vi "LV_n_UDP_clients.vi"() -> ()   [LabVIEW 2020]
panel:
  in  "Open Multi Ports":bool
  in  "Send Test Image":bool
  in  "h":i32=10 min=1 max=5000 step=1
  in  "w":i32=1 min=1 max=5000 step=1
  out "Elaps ms":u32
  in  "Send Image":bool
  out "Path to Python script":path
  in  "Stop":bool
  out "Answer":string
  in  "Ping":bool
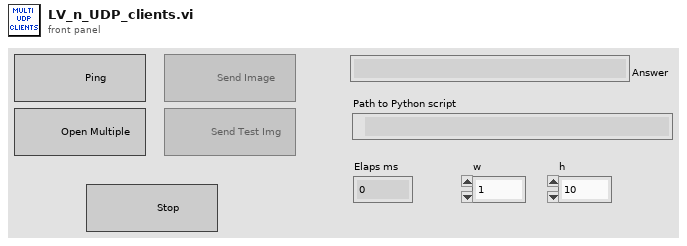
[diagram p1: front panel]
types:
  T1 = enum8{"Enabled", "Disabled", "Disabled and Grayed Out"}
  T2 = typedef "Image Type" = u32
  T3 = typedef "IMAQ Image.ctl" = refnum<image>
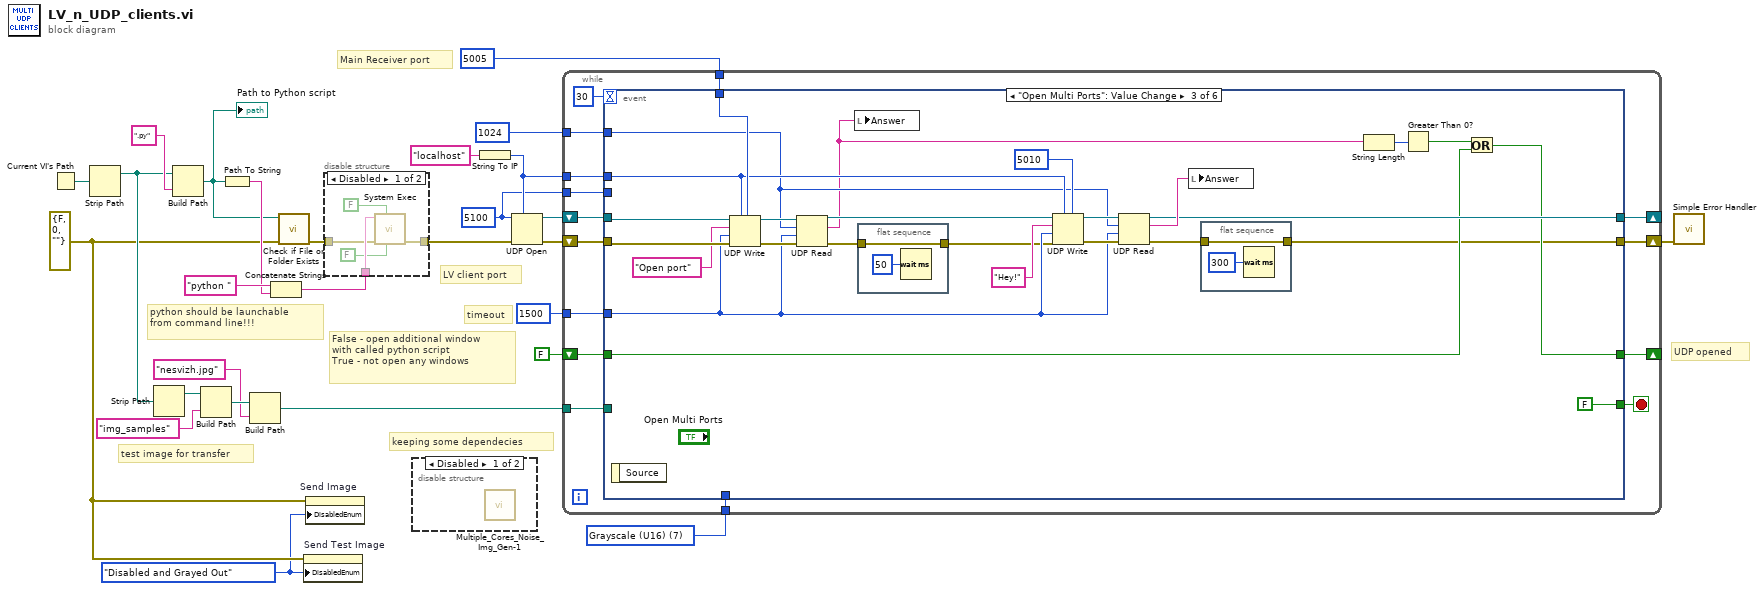
[diagram p0: block diagram]
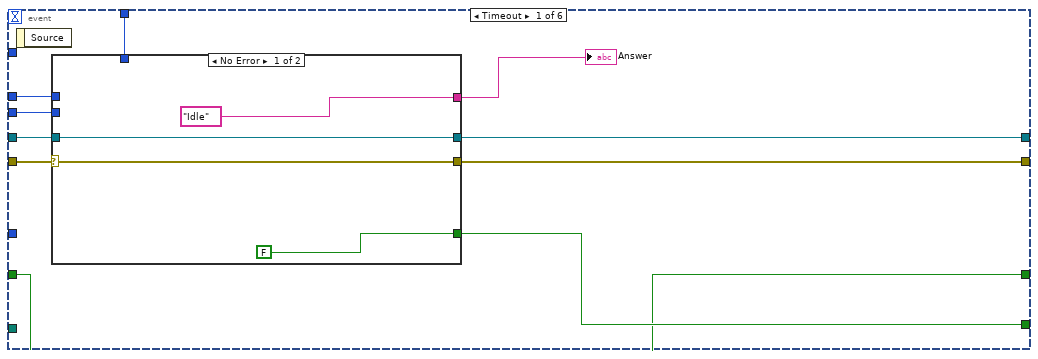
[diagram p4: hidden frame]
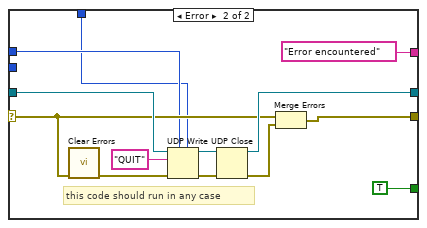
[diagram p5: hidden frame]
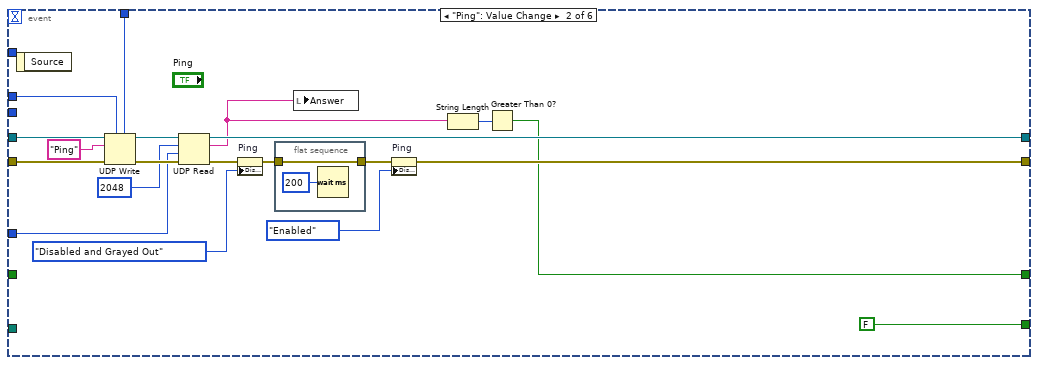
[diagram p6: hidden frame]
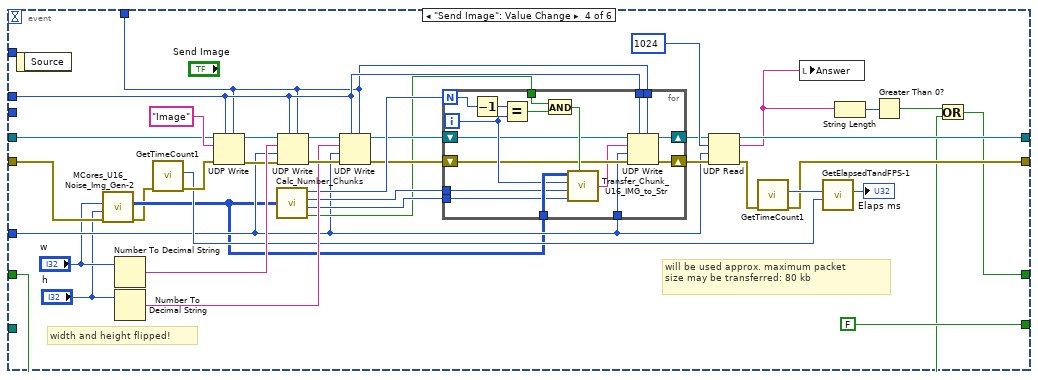
[diagram p7: hidden frame]
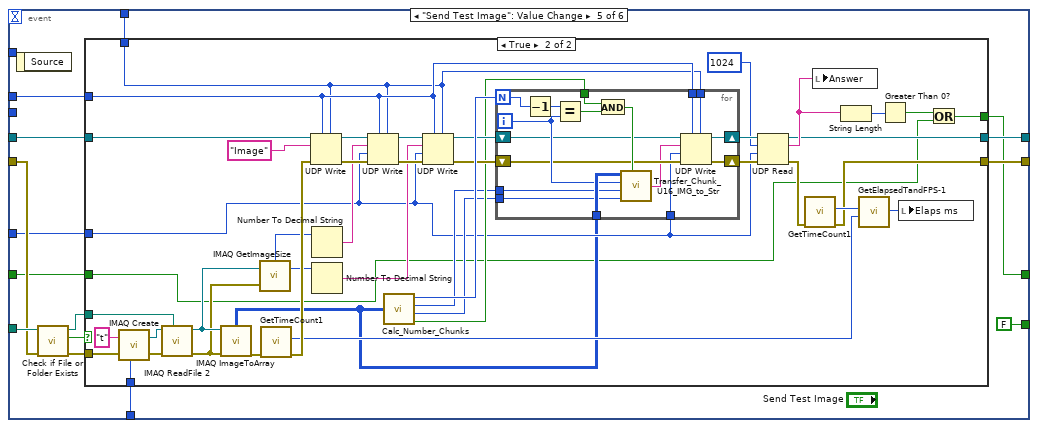
[diagram p8: hidden frame]
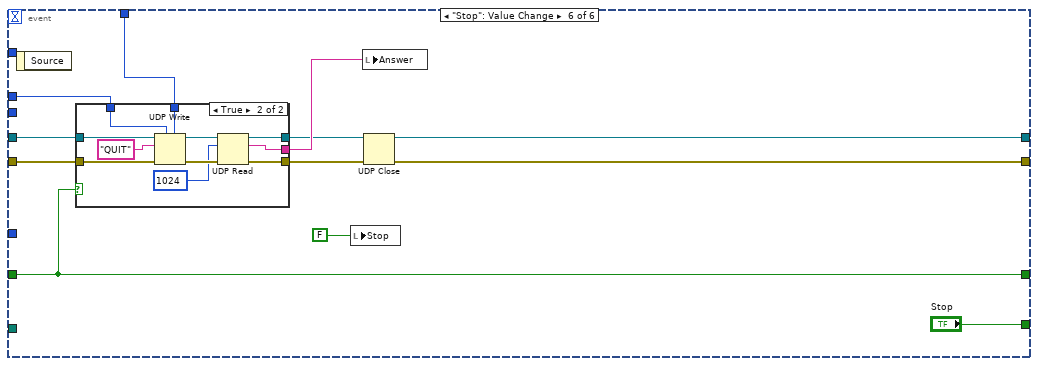
[diagram p10: hidden frame]
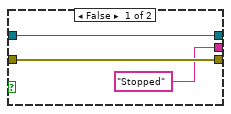
[diagram p11: hidden frame]
diagram:
  w3 = T1."Disabled and Grayed Out" ("Disabled")
  w5 = T2 7 items=["Grayscale (U8)", "Grayscale (I16)", "Grayscale (SGL)", "Complex (CSG)", "RGB (U32)", "HSL (U32)", "RGB (U64)", "Grayscale (U16)"] ("Image Type")
  w14 = u16 5100 ("remote port or service name")
  w4 = errorcluster {"status"=FALSE, "code"=0, "source"=""} ("error in (no error)")
  # "UDP opened"
  # "test image for transfer"
  # "keeping some dependecies"
  # "timeout"
  # "Main Receiver port"
  # "LV client port"
  # "False - open additional window\nwith called python script\nTrue - not open any windows"
  # "python should be launchable \nfrom command line!!!"
  n1 = Current VI's Path() -> (path=w26:path)
  n2 = Strip Path(path=w26) -> (stripped path=w11:path)  [unwired: 1 out]
  n3 = Strip Path(path=w11) -> (stripped path=w10:path)  [unwired: 1 out]
  n4 = Build Path(base path=w11, name or relative path=".py" ("string")) -> (appended path=w21:path)
  "Path to Python script" <- w21
  n5 = Build Path(base path=w10, name or relative path="img_samples" ("string")) -> (appended path=w8:path)
  n6 = Path To String(path=w21) -> (string=w22:string)
  n7 = Build Path(base path=w8, name or relative path="nesvizh.jpg" ("string")) -> (appended path=w6:path)
  n8 = Concatenate Strings("python " ("command line"), w22) -> (w24:string)
  n9 = call <vilib>:"Check if File or Folder Exists.vi"("error in (no error)"=w4, "path"=w21) -> ("error out"=w20:errorcluster)  [unwired: 7 in, 2 out]
  n10 = property on="Send Test Image" class="Bool"(error in=w4, "DisabledEnum"=w3) -> ()  [unwired: 1 in, 2 out]
  n11 = property on="Send Image" class="Bool"(error in=w4, "DisabledEnum"=w3) -> ()  [unwired: 1 in, 2 out]
  n12 = disable-structure shown="Disabled" {
    disable-tunnel: w24 -> [w32 _]
    disable-tunnel: [w31 w33] -> w19
    disable-tunnel: w20 -> [w29 w33]
    frame Disabled {
      n13 = call <vilib>:"System Exec.vi"("run minimized? (F)"=FALSE, "wait until completion? (T)"=FALSE, "error in (no error)"=w29, "command line"=w32) -> ("error out"=w31:errorcluster)  [unwired: 4 in, 3 out]
    }
    frame Enabled {
    }
  }
  n14 = disable-structure shown="Disabled" {
    frame Disabled {
      n15 = call "Multiple_Cores_Noise_Img_Gen-1.vi"() -> ()  [unwired: 10 in, 2 out]
    }
    frame Enabled {
    }
  }
  n16 = String To IP(1:"localhost" ("address")) -> (0:w15:u32)
  n17 = UDP Open(7:w15, 8:w19, 11:w14) -> (port=w17:refnum<k16>, 0:w18:errorcluster)  [unwired: 2 in, 1 out]
  n18 = while {
    shift-right: [w45] -> _
    shift-left: w17 -> [w46]
    shift-right: [w43] -> w27
    shift-left: w18 -> [w47]
    tunnel: w15 -> [w41]
    tunnel: w14 -> [w42]
    tunnel: u16 5005 ("remote port or service name") -> [w40]
    tunnel: 1500 -> [w39]
    tunnel: w6 -> [w38]
    tunnel: w5 -> [w37]
    shift-right: [w35] -> _
    shift-left: FALSE -> [w36]
    tunnel: 1024 -> [w34]
    stop <- w44 stop-if-true
    n19 = event shown="[2] \"Open Multi Ports\": Value Change" {
      selector: _ -> [_ _ _ _ _ _]
      dyn-events: _ -> [_ _ _ _ _ _]
      timeout: 30 -> [_ _ _ _ _ _]
      tunnel: [w54 FALSE ("Stop") FALSE ("Stop") FALSE ("Stop") FALSE ("Stop") "Stop"] -> w44
      tunnel: w47 -> [w58 w89 w123 w137 w195 w268]
      tunnel: w46 -> [w57 w88 w122 w164 w190 w269]
      tunnel: [w56 w84 w108 w158 w185 w270] -> w45
      tunnel: [w55 w91 w100 w150 w186 w271] -> w43
      tunnel: w42 -> [w52 _ _ _ _ _]
      tunnel: w41 -> [w51 w81 w116 w139 w189 w264]
      tunnel: w40 -> [w50 w80 w120 w138 w188 w263]
      tunnel: w39 -> [_ w79 w111 w140 w187 _]
      tunnel: w38 -> [_ _ _ _ w196 _]
      tunnel: w37 -> [_ _ _ _ w191 _]
      tunnel: w36 -> [w49 _ w105 w129 w183 w262]
      tunnel: [w49 w76 w103 w128 w184 w262] -> w35
      tunnel: w34 -> [_ _ w110 _ _ _]
      event Timeout {
        n20 = event-data() -> ()  [unwired: 1 in, 1 out]
        n21 = case shown="No Error" w58 {
          selector: w58 -> [w61 w70]
          tunnel: [w62 w73] -> w56
          tunnel: w57 -> [w62 w72]
          tunnel: [w61 w71] -> w55
          tunnel: [FALSE ("Stop") TRUE ("Stop")] -> w54
          tunnel: ["Idle" ("Answer") "Error encountered" ("Answer")] -> w53
          tunnel: w52 -> [_ _]
          tunnel: w51 -> [_ w69]
          tunnel: w50 -> [_ w68]
          frame No Error {
          }
          frame Error {
            # "this code should run in any case"
            n22 = call <vilib>:"Clear Errors.vi"("error in (no error)"=w70) -> ("error out"=w67:errorcluster)  [unwired: 5 in, 1 out]
            n23 = UDP Write(address=w69, port or service name=w68, connection ID=w72, data in="QUIT", 8:w67) -> (error out=w66:errorcluster, 3:w64:refnum<k16>)  [unwired: 1 in]
            n24 = UDP Close(connection ID=w64, 8:w66) -> (connection ID out=w73:refnum<k16>, error out=w63:errorcluster)
            n25 = Merge Errors(w70, w63) -> (w71:errorcluster)
          }
        }
        "Answer" <- w53
      }
      event "Ping": Value Change {
        n26 = event-data() -> ()  [unwired: 1 in, 1 out]
        n27 = UDP Write(address=w81, port or service name=w80, connection ID=w88, data in="Ping", 8:w89) -> (error out=w86:errorcluster, 3:w85:refnum<k16>)  [unwired: 1 in]
        n28 = UDP Read(connection ID=w85, max size (548)=2048 ("bytes to read"), timeout ms (25000)=w79, 8:w86) -> (data out=w78:string, error out=w83:errorcluster, 3:w84:refnum<k16>)  [unwired: 2 out]
        n29 = property on="Ping" class="Bool"(error in=w83, "DisabledEnum"=T1."Disabled and Grayed Out" ("Disabled")) -> (error out=w94:errorcluster)  [unwired: 1 in, 1 out]
        n30 = flat-sequence {
          tunnel: w94 -> [w96]
          tunnel: [w96] -> w92
          frame #0 {
            n31 = Wait (ms)(milliseconds to wait=u32 200) -> ()  [unwired: 1 out]
          }
        }
        n32 = local write "Answer"(w78) -> ()
        n33 = property on="Ping" class="Bool"(error in=w92, "DisabledEnum"=T1."Enabled" ("Disabled")) -> (error out=w91:errorcluster)  [unwired: 1 in, 1 out]
        n34 = String Length(string=w78) -> (length=w77:i32)
        n35 = Greater Than 0?(x=w77) -> (x > 0?=w76:bool)
      }
      event "Open Multi Ports": Value Change {
        n36 = event-data() -> ()  [unwired: 1 in, 1 out]
        n37 = UDP Write(address=w116, port or service name=w120, connection ID=w122, data in="Open port", 8:w123, 9:w111) -> (error out=w118:errorcluster, 3:w119:refnum<k16>)
        n38 = UDP Read(connection ID=w119, max size (548)=w110, timeout ms (25000)=w111, 8:w118) -> (data out=w106:string, error out=w99:errorcluster, 3:w117:refnum<k16>)  [unwired: 2 out]
        n39 = local write "Answer"(w106) -> ()
        n40 = flat-sequence {
          tunnel: w99 -> [w124]
          tunnel: [w124] -> w98
          frame #0 {
            n41 = Wait (ms)(milliseconds to wait=u32 50) -> ()  [unwired: 1 out]
          }
        }
        n42 = UDP Write(address=w116, port or service name=u16 5010, connection ID=w117, data in="Hey!", 8:w98, 9:w111) -> (error out=w112:errorcluster, 3:w113:refnum<k16>)
        n43 = UDP Read(connection ID=w113, max size (548)=w110, timeout ms (25000)=w111, 8:w112) -> (data out=w109:string, error out=w101:errorcluster, 3:w108:refnum<k16>)  [unwired: 2 out]
        n44 = local write "Answer"(w109) -> ()
        n45 = flat-sequence {
          tunnel: w101 -> [w126]
          tunnel: [w126] -> w100
          frame #0 {
            n46 = Wait (ms)(milliseconds to wait=u32 300) -> ()  [unwired: 1 out]
          }
        }
        n47 = String Length(string=w106) -> (length=w107:i32)
        n48 = Greater Than 0?(x=w107) -> (x > 0?=w104:bool)
        n49 = Or(x=w104, y=w105) -> (x .or. y?=w103:bool)
      }
      event "Send Image": Value Change {
        # "width and height flipped!"
        # "will be used approx. maximum packet \nsize may be transferred: 80 kb"
        n50 = event-data() -> ()  [unwired: 1 in, 1 out]
        n51 = call "MCores_U16_Noise_Img_Gen-2.vi"("error IN"=w137, "[IN] Width"="h", "[IN] Height"="w") -> ("error OUT"=w135:errorcluster, "[OUT] U16 Pixel Img"=w136:u16[][])  [unwired: 7 in]
        n52 = Number To Decimal String(number="w") -> (decimal integer string=w160:string)  [unwired: 1 in]
        n53 = Number To Decimal String(number="h") -> (decimal integer string=w157:string)  [unwired: 1 in]
        n54 = call "GetTimeCount1.vi"("error IN"=w135) -> ("error OUT"=w154:errorcluster, "[OUT] Timer Count"=w151:u32)  [unwired: 9 in]
        n55 = UDP Write(address=w139, port or service name=w138, connection ID=w164, data in="Image", 8:w154) -> (error out=w155:errorcluster, 3:w156:refnum<k16>)  [unwired: 1 in]
        n56 = call "Calc_Number_Chunks.vi"("[IN] U16 Pixel Img"=w136) -> ("[OUT] Number of chunks"=w147:i32, "[OUT] # rows single transfer"=w146:i32, "[OUT] # rows last transfer"=w145:i32, "[OUT] Not-equal last transfer"=w141:bool)
        n57 = UDP Write(address=w139, port or service name=w138, connection ID=w156, data in=w160, 8:w155, 9:w140) -> (error out=w163:errorcluster, 3:w162:refnum<k16>)
        n58 = UDP Write(address=w139, port or service name=w138, connection ID=w162, data in=w157, 8:w163, 9:w140) -> (error out=w143:errorcluster, 3:w144:refnum<k16>)
        n59 = for {
          N: w147 -> [w182]
          shift-right: [w172] -> w148
          shift-left: w143 -> [w173]
          tunnel: w136 -> [w180]
          tunnel: w146 -> [w175]
          tunnel: w145 -> [w174]
          shift-right: [w171] -> w142
          shift-left: w144 -> [w170]
          tunnel: w141 -> [w177]
          tunnel: w140 -> [w168]
          tunnel: w139 -> [w167]
          tunnel: w138 -> [w166]
          i -> [w178]
          n60 = Decrement(x=w182) -> (x-1=w181:i32)
          n61 = Equal?(x=w181, y=w178) -> (x = y?=w176:bool)
          n62 = And(x=w177, y=w176) -> (x .and. y?=w179:bool)
          n63 = call "Transfer_Chunk_U16_IMG_to_Str.vi"("[IN] U16 Pixel Img"=w180, "[IN] # of chunk"=w178, "[IN] # rows single transfer"=w175, "[IN] # rows last transfer"=w174, "[IN] Use remained rows"=w179) -> ("[OUT] Converted String"=w169:string)
          n64 = UDP Write(address=w167, port or service name=w166, connection ID=w170, data in=w169, 8:w173, 9:w168) -> (error out=w172:errorcluster, 3:w171:refnum<k16>)
        }
        n65 = UDP Read(connection ID=w142, max size (548)=1024 ("bytes to read"), timeout ms (25000)=w140, 8:w148) -> (data out=w131:string, error out=w153:errorcluster, 3:w158:refnum<k16>)  [unwired: 2 out]
        n66 = call "GetTimeCount1.vi"("error IN"=w153) -> ("error OUT"=w150:errorcluster, "[OUT] Timer Count"=w152:u32)  [unwired: 9 in]
        n67 = local write "Answer"(w131) -> ()
        n68 = call "GetElapsedTandFPS-1.vi"("[IN] Timer Count Before ALL [ms]"=w151, "[IN] Timer Count After ALL [ms]"=w152) -> ("[OUT] Elapsed time [ms]"=→"Elaps ms":u32)  [unwired: 3 in, 2 out]
        n69 = String Length(string=w131) -> (length=w132:i32)
        n70 = Greater Than 0?(x=w132) -> (x > 0?=w130:bool)
        n71 = Or(x=w130, y=w129) -> (x .or. y?=w128:bool)
      }
      event "Send Test Image": Value Change {
        n72 = event-data() -> ()  [unwired: 1 in, 1 out]
        n73 = call <vilib>:"Check if File or Folder Exists.vi"("error in (no error)"=w195, "path"=w196) -> ("error out"=w194:errorcluster, "file or folder exists?"=w193:bool, "dup path"=w192:path)  [unwired: 7 in]
        n74 = case shown="True" w193 {
          tunnel: w194 -> [w199 w244]
          tunnel: w192 -> [_ w239]
          tunnel: w191 -> [_ w243]
          tunnel: w190 -> [w200 w237]
          tunnel: w189 -> [_ w218]
          tunnel: w188 -> [_ w217]
          tunnel: w187 -> [_ w214]
          tunnel: [w199 w208] -> w186
          tunnel: [w200 w203] -> w185
          tunnel: [w198 w202] -> w184
          tunnel: w183 -> [w198 w201]
          frame False {
          }
          frame True {
            n75 = call "IMAQ Create"("Image Name"="t", "Image Type"=w243, "error in (no error)"=w244) -> ("New Image"=w240:T3, "error out"=w241:errorcluster)  [unwired: 2 in]
            n76 = call "IMAQ ReadFile 2"("File Path"=w239, "error in (no error)"=w241, "Image"=w240) -> ("error out"=w233:errorcluster, "Image Out"=w234:T3)  [unwired: 4 in, 3 out]
            n77 = call "IMAQ ImageToArray"("error in (no error)"=w233, "Image"=w234) -> ("error out"=w238:errorcluster, "Image Pixels (U8)"=w207:u8[][])  [unwired: 2 in, 3 out]
            n78 = call "IMAQ GetImageSize"("Image"=w234, "error in (no error)"=w233) -> ("Y Resolution"=w231:i32, "X Resolution"=w232:i32)  [unwired: 2 in, 1 out]
            n79 = call "GetTimeCount1.vi"("error IN"=w238) -> ("error OUT"=w236:errorcluster, "[OUT] Timer Count"=w211:u32)  [unwired: 9 in]
            n80 = UDP Write(address=w218, port or service name=w217, connection ID=w237, data in="Image", 8:w236) -> (error out=w230:errorcluster, 3:w229:refnum<k16>)  [unwired: 1 in]
            n81 = Number To Decimal String(number=w232) -> (decimal integer string=w228:string)  [unwired: 1 in]
            n82 = Number To Decimal String(number=w231) -> (decimal integer string=w225:string)  [unwired: 1 in]
            n83 = UDP Write(address=w218, port or service name=w217, connection ID=w229, data in=w228, 8:w230, 9:w214) -> (error out=w226:errorcluster, 3:w227:refnum<k16>)
            n84 = call "Calc_Number_Chunks.vi"("[IN] U16 Pixel Img"=w207) -> ("[OUT] Number of chunks"=w224:i32, "[OUT] # rows single transfer"=w220:i32, "[OUT] # rows last transfer"=w219:i32, "[OUT] Not-equal last transfer"=w221:bool)
            n85 = UDP Write(address=w218, port or service name=w217, connection ID=w227, data in=w225, 8:w226, 9:w214) -> (error out=w222:errorcluster, 3:w223:refnum<k16>)
            n86 = for {
              N: w224 -> [w261]
              shift-right: [w251] -> w216
              shift-left: w222 -> [w252]
              tunnel: w207 -> [w259]
              tunnel: w220 -> [w254]
              tunnel: w219 -> [w253]
              shift-right: [w250] -> w215
              shift-left: w223 -> [w249]
              tunnel: w221 -> [w256]
              tunnel: w214 -> [w247]
              tunnel: w218 -> [w246]
              tunnel: w217 -> [w245]
              i -> [w257]
              n87 = Decrement(x=w261) -> (x-1=w260:i32)
              n88 = Equal?(x=w260, y=w257) -> (x = y?=w255:bool)
              n89 = And(x=w256, y=w255) -> (x .and. y?=w258:bool)
              n90 = call "Transfer_Chunk_U16_IMG_to_Str.vi"("[IN] U16 Pixel Img"=w259, "[IN] # of chunk"=w257, "[IN] # rows single transfer"=w254, "[IN] # rows last transfer"=w253, "[IN] Use remained rows"=w258) -> ("[OUT] Converted String"=w248:string)
              n91 = UDP Write(address=w246, port or service name=w245, connection ID=w249, data in=w248, 8:w252, 9:w247) -> (error out=w251:errorcluster, 3:w250:refnum<k16>)
            }
            n92 = UDP Read(connection ID=w215, max size (548)=1024 ("bytes to read"), timeout ms (25000)=w214, 8:w216) -> (data out=w205:string, error out=w213:errorcluster, 3:w203:refnum<k16>)  [unwired: 2 out]
            n93 = call "GetTimeCount1.vi"("error IN"=w213) -> ("error OUT"=w208:errorcluster, "[OUT] Timer Count"=w212:u32)  [unwired: 9 in]
            n94 = local write "Answer"(w205) -> ()
            n95 = String Length(string=w205) -> (length=w206:i32)
            n96 = call "GetElapsedTandFPS-1.vi"("[IN] Timer Count Before ALL [ms]"=w211, "[IN] Timer Count After ALL [ms]"=w212) -> ("[OUT] Elapsed time [ms]"=w209:u32)  [unwired: 3 in, 2 out]
            n97 = Greater Than 0?(x=w206) -> (x > 0?=w204:bool)
            n98 = local write "Elaps ms"(w209) -> ()
            n99 = Or(x=w204, y=w201) -> (x .or. y?=w202:bool)
          }
        }
      }
      event "Stop": Value Change {
        n100 = event-data() -> ()  [unwired: 1 in, 1 out]
        n101 = case shown="True" w262 {
          tunnel: w269 -> [w276 w287]
          tunnel: w268 -> [w275 w286]
          tunnel: [w275 w282] -> w267
          tunnel: ["Stopped" ("data out") w281] -> w266
          tunnel: [w276 w280] -> w265
          tunnel: w264 -> [_ w278]
          tunnel: w263 -> [_ w277]
          frame False {
          }
          frame True {
            n102 = UDP Write(address=w278, port or service name=w277, connection ID=w287, data in="QUIT", 8:w286) -> (error out=w283:errorcluster, 3:w284:refnum<k16>)  [unwired: 1 in]
            n103 = UDP Read(connection ID=w284, max size (548)=1024 ("bytes to read"), 8:w283) -> (data out=w281:string, error out=w282:errorcluster, 3:w280:refnum<k16>)  [unwired: 1 in, 2 out]
          }
        }
        n104 = local write "Stop"(FALSE ("Stop")) -> ()
        n105 = local write "Answer"(w266) -> ()
        n106 = UDP Close(connection ID=w265, 8:w267) -> (connection ID out=w270:refnum<k16>, error out=w271:errorcluster)
      }
    }
  }
  n107 = call <vilib>:"Simple Error Handler.vi"("error in (no error)"=w27) -> ()  [unwired: 4 in, 5 out]
